vi "Query Questionable Data Register.vi"(8 "error in (no error)":errorcluster, 11 "VISA resource name":refnum<visa-resource-name>) -> (0 "error out":errorcluster, 1 "Questionable Data Message":string, 3 "VISA resource name out":refnum<visa-resource-name>)   [LabVIEW 2018, in "Agilent 34401.lvlib"]
doc: "Queries the event register for the Questionable Data Register group. Essentially, it is used to observe possible invalid results. For example, if the set sample interval is less than the minimum sample interval, the questionable data register will be set. This VI will then return the corresponding warning(s)."
uses:
  <instrlib>/Agilent 34401/Agilent 34401.lvlib
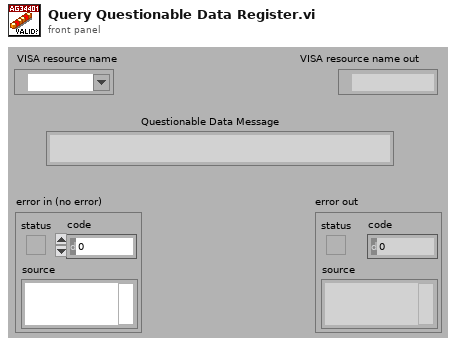
[diagram p1: front panel]
types:
  T1 = cluster{"Boolean array[0]":bool, "Boolean array[1]":bool, "Boolean array[2]":bool, "Boolean array[3]":bool, "Boolean array[4]":bool, "Boolean array[5]":bool, "Boolean array[6]":bool, "Boolean array[7]":bool, "Boolean array[8]":bool, "Boolean array[9]":bool, "Boolean array[10]":bool, "Boolean array[11]":bool, "Boolean array[12]":bool, "Boolean array[13]":bool, "Boolean array[14]":bool, "Boolean array[15]":bool}
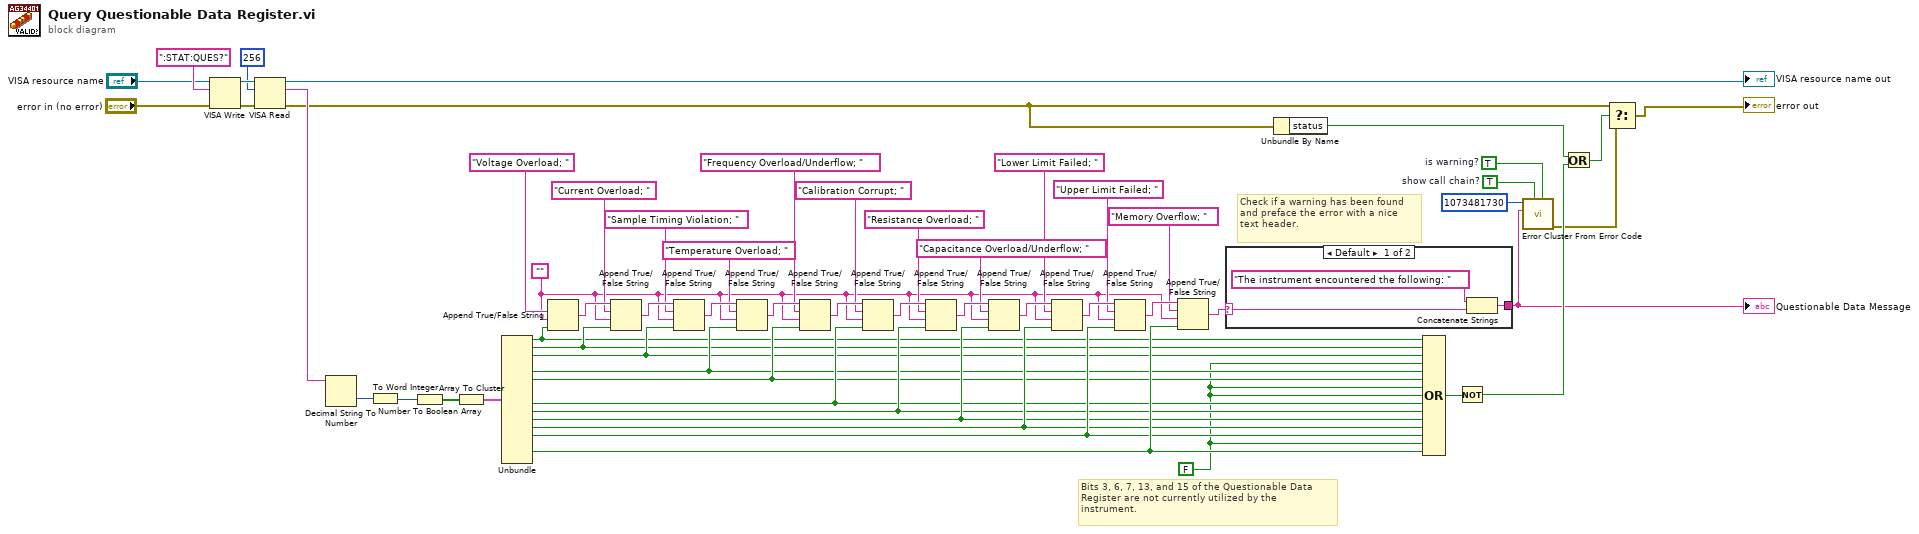
[diagram p0: block diagram]
diagram:
  w4 = TRUE  # is warning?
  w5 = TRUE  # show call chain?
  w14 = FALSE
  w28 = ""
  # "Check if a warning has been found and preface the error with a nice text header."
  # "Bits 3, 6, 7, 13, and 15 of the Questionable Data Register are not currently utilized by the instrument."
  n1 = VISA Write(VISA resource name="VISA resource name", write buffer=":STAT:QUES?", error in (no error)="error in (no error)") -> (VISA resource name out=w56:refnum<visa-resource-name>, error out=w57:errorcluster)  [unwired: 1 out]
  n2 = VISA Read(VISA resource name=w56, byte count=u32 256, error in (no error)=w57) -> (VISA resource name out=→"VISA resource name out":refnum<visa-resource-name>, read buffer=w54:string, error out=w8:errorcluster)  [unwired: 1 out]
  n3 = Decimal String To Number(string=w54) -> (number=w51:i32)  [unwired: 2 in, 1 out]
  n4 = To Word Integer(number=w51) -> (16bit integer=w52:i16)
  n5 = Number To Boolean Array(number=w52) -> (Boolean array=w53:bool[])
  n6 = Array To Cluster(array=w53) -> (cluster=w50:T1)
  n7 = Unbundle(w50) -> ("Boolean array[0]"=w15:bool, "Boolean array[1]"=w16:bool, "Boolean array[2]"=w17:bool, "Boolean array[4]"=w18:bool, "Boolean array[5]"=w19:bool, "Boolean array[8]"=w20:bool, "Boolean array[9]"=w21:bool, "Boolean array[10]"=w22:bool, "Boolean array[11]"=w23:bool, "Boolean array[12]"=w24:bool, "Boolean array[14]"=w25:bool)  [unwired: 5 out]
  n8 = Append True/False String(1:w15, 2:w28, 3:"Voltage Overload; " ("true string")) -> (0:w49:string)  [unwired: 1 in]
  n9 = Append True/False String(1:w16, 2:w28, 3:"Current Overload; " ("true string"), 4:w49) -> (0:w48:string)
  n10 = Append True/False String(1:w17, 2:w28, 3:"Sample Timing Violation; " ("true string"), 4:w48) -> (0:w47:string)
  n11 = Append True/False String(1:w18, 2:w28, 3:"Temperature Overload; " ("true string"), 4:w47) -> (0:w46:string)
  n12 = Append True/False String(1:w19, 2:w28, 3:"Frequency Overload/Underflow; " ("true string"), 4:w46) -> (0:w45:string)
  n13 = Append True/False String(1:w20, 2:w28, 3:"Calibration Corrupt; " ("true string"), 4:w45) -> (0:w44:string)
  n14 = Append True/False String(1:w21, 2:w28, 3:"Resistance Overload; " ("true string"), 4:w44) -> (0:w43:string)
  n15 = Append True/False String(1:w22, 2:w28, 3:"Capacitance Overload/Underflow; " ("true string"), 4:w43) -> (0:w42:string)
  n16 = Append True/False String(1:w23, 2:w28, 3:"Lower Limit Failed; " ("true string"), 4:w42) -> (0:w41:string)
  n17 = Append True/False String(1:w24, 2:w28, 3:"Upper Limit Failed; " ("true string"), 4:w41) -> (0:w40:string)
  n18 = Append True/False String(1:w25, 2:w28, 3:"Memory Overflow; " ("true string"), 4:w40) -> (0:w2:string)
  n19 = case shown="Default" w2 {
    selector: w2 -> [w60 w62]
    tunnel: [w59 w62] -> w1
    frame Default {
      n20 = Concatenate Strings("The instrument encountered the following: " ("true string"), w60) -> (w59:string)
    }
    frame "" {
    }
  }
  "Questionable Data Message" <- w1
  n21 = Unbundle By Name(w8) -> ("status"=w11:bool)
  n22 = Compound Arithmetic op=OR(w15, w16, w17, w14, w18, w19, w14, w14, w20, w21, w22, w23, w24, w14, w25) -> (w13:bool)
  n23 = Not(x=w13) -> (.not. x?=w12:bool)
  n24 = call <vilib>:"Error Cluster From Error Code.vi"("is warning? (False)"=w4, "show call chain? (False)"=w5, "error message (\"\")"=w1, "error code (0)"=1073481730 ("t")) -> ("error out"=w7:errorcluster)  [unwired: 5 in]
  n25 = Or(x=w11, y=w12) -> (x .or. y?=w10:bool)
  n26 = Select(t=w8, s=w10, f=w7) -> (s? t:f=→"error out":errorcluster)
